vi "Conversor_2.vi"() -> ()   [LabVIEW 2016]
panel:
  out "output cluster":T1
  in  "Z":bool
  in  "Y":bool
  in  "X":bool
  in  "W":bool
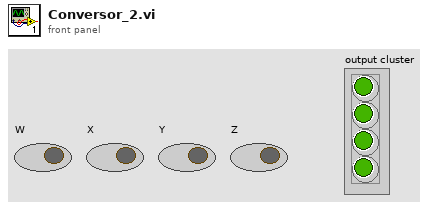
[diagram p1: front panel]
types:
  T1 = cluster{"Boolean":bool, "Boolean":bool, "Boolean":bool, "Boolean":bool}
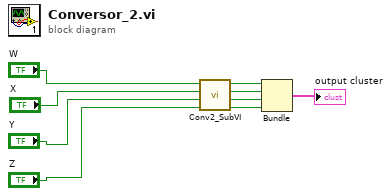
[diagram p0: block diagram]
diagram:
  n1 = call "Conv2_SubVI.vi"("Z"="Z", "Y"="Y", "X"="X", "W"="W") -> ("D"=w2:bool, "C"=w3:bool, "B"=w4:bool, "A"=w5:bool)
  n2 = Bundle("A"=w5, "B"=w4, "C"=w3, "D"=w2) -> (→"output cluster":cluster{"A":bool, "B":bool, "C":bool, "D":bool})  [unwired: 1 in]
